vi "Get Attributes.vi"(8 "error in (no error)":errorcluster, 11 "For Loop Dialog in":refnum<class "Test Step Dialog.lvclass">) -> (0 "error out":errorcluster, 3 "For Loop Dialog out":refnum<class "Test Step Dialog.lvclass">)   [LabVIEW 2017, in "Test Step Dialog.lvclass"]
uses:
  Test Step Dialog.lvclass
  D:/Test-executive-builder/Source/Test Executive Builder Dialogs/ITest Executive Builder Dialog/ITest Executive Builder Dialog.lvclass
  ITest Executive Builder Dialog/ITest Executive Builder Dialog.lvclass/ITest Executive Builder Dialog.ctl
  Test Step Dialog.lvclass/Test Step Dialog.ctl
  210526c6-8347-4f83-98d4-bf6ff259764b.vi
  6281bc39-4b1f-4fa0-b6e5-3275a081bde5.vi
  37054371-845d-43d0-a581-1ea5269a3f09.vi
  <vilib>/Utility/error.llb/Clear Errors.vi
  <vilib>/gpm_packages/@cs/test-executive/Source/Test Executive/ITestExecutive/ITest Executive.lvclass
  Data Type Handler/Test Executive Builder Data Type Handler.lvclass
  ITest Executive Builder Dialog/ITest Executive Builder Dialog.lvclass
  <vilib>/gpm_packages/@cs/test-executive/Source/Test Executive/TestExecutive Ref/TestExecutive Ref.lvclass
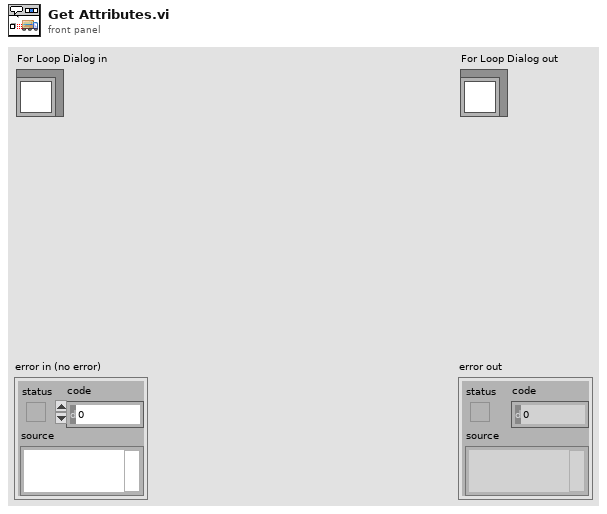
[diagram p1: front panel]
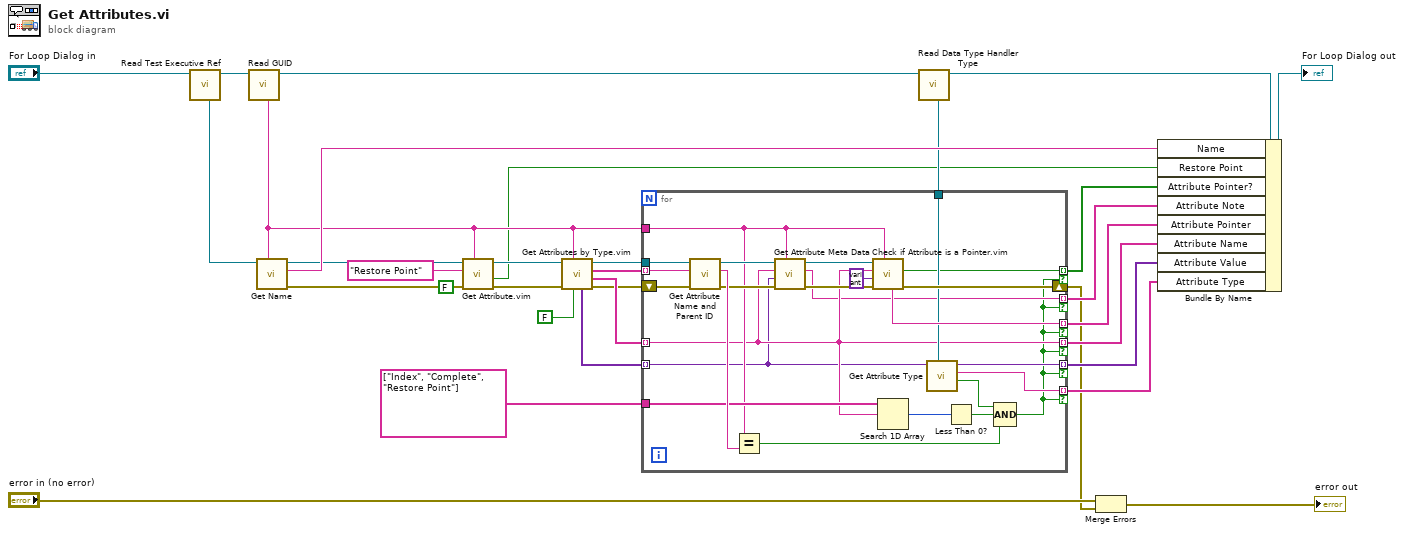
[diagram p0: block diagram]
diagram:
  n1 = call "Read Test Executive Ref.vi"("ITest Executive Builder Dialog in"="For Loop Dialog in") -> ("ITest Executive Builder Dialog out"=w31:refnum<class "Test Step Dialog.lvclass">, "Test Executive Ref"=w28:refnum<data-value>)  [unwired: 9 in]
  n2 = call "Read GUID.vi"("ITest Executive Builder Dialog in"=w31) -> ("ITest Executive Builder Dialog out"=w12:refnum<class "Test Step Dialog.lvclass">, "GUID"=w14:string)  [unwired: 9 in]
  n3 = call <vilib>:"Get Name.vi"("Unique ID"=w14, "Test Executive Ref"=w28) -> ("error out"=w24:errorcluster, "Name"=w30:string, "Test Executive Ref out"=w25:refnum<data-value>)  [unwired: 5 in, 2 out]
  n4 = call "Get Attribute.vim"("ID"=w14, "error in (no error)"=w24, "Type"=FALSE, "Attribute Name"="Restore Point", "Test Executive Ref"=w25) -> ("error out"=w20:errorcluster, "Attribute"=w8:bool, "Test Executive Ref out"=w21:refnum<data-value>)  [unwired: 2 in, 2 out]
  n5 = call "Get Attributes by Type.vim"("Recurse Up List (Default=True)"=FALSE, "ID"=w14, "error in (no error)"=w20, "Test Executive Ref"=w21) -> ("error out"=w15:errorcluster, "Names"=w16:string[], "IDs"=w17:string[], "Test Executive Ref out"=w18:refnum<data-value>, "Attributes"=w13:variant[])  [unwired: 3 in]
  n6 = call "Read Data Type Handler Type.vi"("ITest Executive Builder Dialog in"=w12) -> ("ITest Executive Builder Dialog out"=w11:refnum<class "Test Step Dialog.lvclass">, "Data Type Handler"=w10:refnum<class "Test Executive Builder Data Type Handler.lvclass">)  [unwired: 9 in]
  n7 = for {
    tunnel: w18 -> [w57]
    tunnel: w17 -> [w56] mode=indexing
    tunnel: w16 -> [w37] mode=indexing
    shift-right: [w52] -> w1
    shift-left: w15 -> [w55]
    tunnel: w14 -> [w38]
    tunnel: w13 -> [w36] mode=indexing
    tunnel: [w33] -> w7 mode=indexing if=w34
    tunnel: [w51] -> w6 mode=indexing if=w34
    tunnel: [w37] -> w5 mode=indexing if=w34
    tunnel: w10 -> [w50]
    tunnel: [w48] -> w3 mode=indexing if=w34
    tunnel: [w47] -> w4 mode=indexing if=w34
    tunnel: string[] ["Index", "Complete", "Restore Point"] -> [w46]
    tunnel: [w35] -> w2 mode=indexing if=w34
    n8 = call <vilib>:"Get Attribute Name and Parent ID.vi"("error in (no error)"=w55, "Tag"=w56, "Test Executive Ref"=w57) -> ("error out"=w40:errorcluster, "Parent ID"=w53:string, "Test Executive Ref out"=w42:refnum<data-value>)  [unwired: 5 in, 1 out]
    n9 = Equal?(x=w38, y=w53) -> (x = y?=w43:bool)
    n10 = call <vilib>:"Get Attribute Meta Data.vi"("Unique ID"=w38, "error in (no error)"=w40, "Attribute Type"=w36, "Attribute Name"=w37, "Test Executive Ref"=w42) -> ("error out"=w39:errorcluster, "Meta Data"=w35:string, "Test Executive Ref out"=w41:refnum<data-value>)  [unwired: 3 in, 1 out]
    n11 = call "Check if Attribute is a Pointer.vim"("ID"=w38, "error in (no error)"=w39, "Type"=variant, "Attribute Name"=w37, "Test Executive Ref"=w41) -> ("error out"=w52:errorcluster, "Pointer?"=w33:bool, "Pointer ID"=w51:string)  [unwired: 2 in, 2 out]
    n12 = Search 1D Array(1D array=w46, element=w37) -> (index of element=w45:i32)  [unwired: 1 in]
    n13 = call-dynamic "Get Attribute Type.vi"("Test Executive Builder Data Type Handler in"=w50, "Potential Attribute in"=w36) -> ("Valid Type?"=w49:bool, "Attribute Type"=w48:string, "Potential Attribute out"=w47:variant)  [unwired: 6 in, 1 out]
    n14 = Less Than 0?(x=w45) -> (x < 0?=w44:bool)
    n15 = Compound Arithmetic op=AND(w49, w44, w43) -> (w34:bool)
  }
  n16 = Merge Errors("error in (no error)", w1) -> (→"error out":errorcluster)
  n17 = Bundle By Name(cluster=w11, "Name"=w30, "Restore Point"=w8, "Attribute Pointer?"=w7, "Attribute Note"=w2, "Attribute Pointer"=w6, "Attribute Name"=w5, "Attribute Value"=w4, "Attribute Type"=w3) -> (→"For Loop Dialog out":refnum<class "Test Step Dialog.lvclass">)
